vi "PH_SHS_Analysis.unpack Zernickes.vi"(1 "DIM Service Array":dbl[](array[numeric])) -> (0 "SHS Analyzer Dataset":T1 {"State" items=["no info", "off/false/out", "on/true/in", "Failure", "Alarm", "Status 1", "Status 2", "Status 3"]; "Zernicke Coefficients"."2nd Spherical" scale=-2.0..2.0 scale format="%.2f"; "Zernicke Coefficients"."2nd Coma y" scale=-2.0..2.0 scale format="%.2f"; "Zernicke Coefficients"."2nd Coma x" scale=-2.0..2.0 scale format="%.2f"; "Zernicke Coefficients"."2nd Astig 45°" scale=-2.0..2.0 scale format="%.2f"; "Zernicke Coefficients"."2nd Astig 0°" scale=-2.0..2.0 scale format="%.2f"; "Zernicke Coefficients"."Trefoil 30°" scale=-2.0..2.0 scale format="%.2f"; "Zernicke Coefficients"."Trefoil 0°" scale=-2.0..2.0 scale format="%.2f"; "Zernicke Coefficients"."Spherical" scale=-2.0..2.0 scale format="%.2f"; "Zernicke Coefficients"."Coma y" scale=-2.0..2.0 scale format="%.2f"; "Zernicke Coefficients"."Coma x" scale=-2.0..2.0 scale format="%.2f"; "Zernicke Coefficients"."Astig 45°" scale=-2.0..2.0 scale format="%.2f"; "Zernicke Coefficients"."Astig 0°" scale=-2.0..2.0 scale format="%.2f"; "Zernicke Coefficients"."Defocus" scale=-2.0..2.0 scale format="%.2f"; "Zernicke Coefficients"."Tilt y" scale=-2.0..2.0 scale format="%.2f"; "Zernicke Coefficients"."Tilt x" scale=-2.0..2.0 scale format="%.2f"})   [LabVIEW 2014, in "PH_SHS_Analysis.lvlib"]
doc: "This VI unpacks the DIM service Data \"<SHS Anaylzer Instance>_Zernikes\" published by a SHS Analyzer."
uses:
  PH_SHS_Analysis.lvlib
  PH_SHS_Analysis.Zernike Dataset.ctl
  PH_StatusHandler/PH_StatusHandler.Status.ctl
  PH_SHS_Analysis.Zernike Coefficients.ctl
  PH_StatusHandler/PH_StatusHandler.lvlib
panel:
  in  "SHS Analyzer Dataset Dummy":T1 {"State" items=["no info", "off/false/out", "on/true/in", "Failure", "Alarm", "Status 1", "Status 2", "Status 3"]; "Zernicke Coefficients"."2nd Spherical" scale=-2.0..2.0 scale format="%.2f"; "Zernicke Coefficients"."2nd Coma y" scale=-2.0..2.0 scale format="%.2f"; "Zernicke Coefficients"."2nd Coma x" scale=-2.0..2.0 scale format="%.2f"; "Zernicke Coefficients"."2nd Astig 45°" scale=-2.0..2.0 scale format="%.2f"; "Zernicke Coefficients"."2nd Astig 0°" scale=-2.0..2.0 scale format="%.2f"; "Zernicke Coefficients"."Trefoil 30°" scale=-2.0..2.0 scale format="%.2f"; "Zernicke Coefficients"."Trefoil 0°" scale=-2.0..2.0 scale format="%.2f"; "Zernicke Coefficients"."Spherical" scale=-2.0..2.0 scale format="%.2f"; "Zernicke Coefficients"."Coma y" scale=-2.0..2.0 scale format="%.2f"; "Zernicke Coefficients"."Coma x" scale=-2.0..2.0 scale format="%.2f"; "Zernicke Coefficients"."Astig 45°" scale=-2.0..2.0 scale format="%.2f"; "Zernicke Coefficients"."Astig 0°" scale=-2.0..2.0 scale format="%.2f"; "Zernicke Coefficients"."Defocus" scale=-2.0..2.0 scale format="%.2f"; "Zernicke Coefficients"."Tilt y" scale=-2.0..2.0 scale format="%.2f"; "Zernicke Coefficients"."Tilt x" scale=-2.0..2.0 scale format="%.2f"}
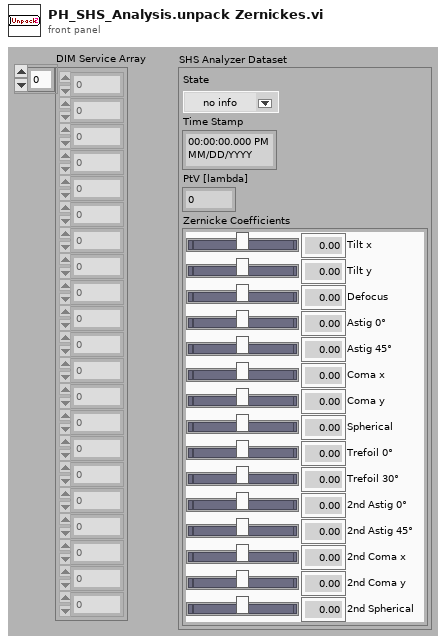
[diagram p1: front panel]
types:
  T1 = typedef "PH_SHS_Analysis.lvlib/PH_SHS_Analysis.Zernike Dataset.ctl" = cluster{"State":T2, "Time Stamp":timestamp, "PtV [lambda]":dbl, "Zernicke Coefficients":T3}
  T2 = typedef "PH_StatusHandler.lvlib/PH_StatusHandler.Status.ctl" = i16
  T3 = typedef "PH_SHS_Analysis.lvlib/PH_SHS_Analysis.Zernike Coefficients.ctl" = cluster{"Tilt x":dbl, "Tilt y":dbl, "Defocus":dbl, "Astig 0°":dbl, "Astig 45°":dbl, "Coma x":dbl, "Coma y":dbl, "Spherical":dbl, "Trefoil 0°":dbl, "Trefoil 30°":dbl, "2nd Astig 0°":dbl, "2nd Astig 45°":dbl, "2nd Coma x":dbl, "2nd Coma y":dbl, "2nd Spherical":dbl}
  T4 = cluster{"DIM Service Array[0]":dbl, "DIM Service Array[1]":dbl, "DIM Service Array[2]":dbl, "DIM Service Array[3]":dbl, "DIM Service Array[4]":dbl, "DIM Service Array[5]":dbl, "DIM Service Array[6]":dbl, "DIM Service Array[7]":dbl, "DIM Service Array[8]":dbl, "DIM Service Array[9]":dbl, "DIM Service Array[10]":dbl, "DIM Service Array[11]":dbl, "DIM Service Array[12]":dbl, "DIM Service Array[13]":dbl, "DIM Service Array[14]":dbl}
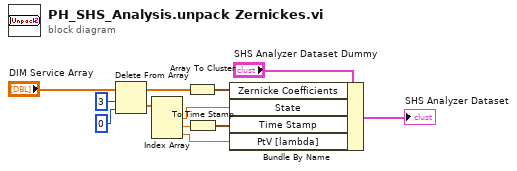
[diagram p0: block diagram]
diagram:
  n1 = Delete From Array(array="DIM Service Array", length=3, index=0) -> (deleted portion=w4:dbl[], array with subset deleted=w6:dbl[])
  n2 = Index Array(array=w4) -> (element #1=w10:dbl, element #2=w8:dbl, element #3=w9:dbl)  [unwired: 3 in]
  n3 = Array To Cluster(array=w6) -> (cluster=w5:T4)
  n4 = To Time Stamp(1:w8) -> (0:w7:timestamp)
  n5 = Bundle By Name(cluster="SHS Analyzer Dataset Dummy", "Zernicke Coefficients"=w5, "State"=w10, "Time Stamp"=w7, "PtV [lambda]"=w9) -> (→"SHS Analyzer Dataset":T1)
